vi "Create.vi"(8 "error in (no error)":errorcluster) -> (0 "error out":errorcluster, 3 "ClientPool out":refnum<class "ClientPool.lvclass">)   [LabVIEW 2020, in "MeasurementLink Measurement Server.lvlib" / "ClientPool.lvclass"]
uses:
  ClientPool.lvclass
  ClientPool.lvclass/ClientPool.ctl
  MeasurementLink Measurement Server.lvlib
  MeasurementLink Discovery Client/MeasurementLink Discovery Client.lvlib
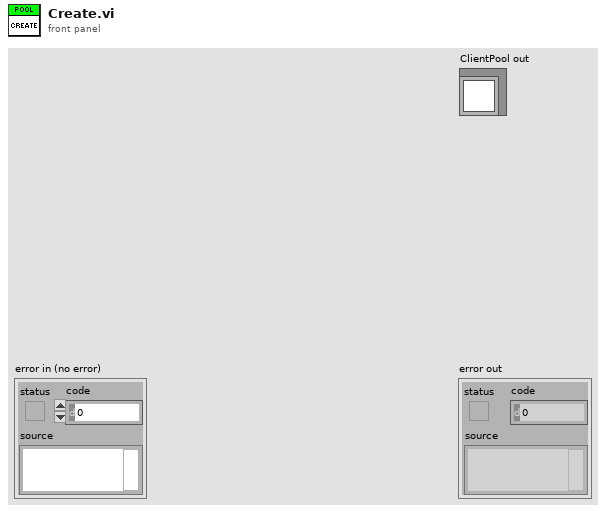
[diagram p1: front panel]
types:
  T1 = typedef "grpc-lvsupport-release.lvlib/grpcId.ctl" = u64
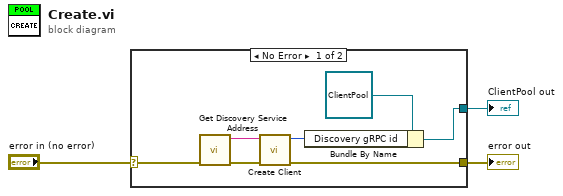
[diagram p0: block diagram]
diagram:
  n1 = case shown="No Error" "error in (no error)" {
    selector: "error in (no error)" -> [w8 w11]
    tunnel: [w7 w11] -> w2
    tunnel: [w9 _] -> w1
    frame No Error {
      n2 = call "Get Discovery Service Address.vi"("error in"=w8) -> ("error out"=w10:errorcluster, "address"=w5:string)  [unwired: 9 in]
      n3 = call "Create Client.vi"("error in"=w10, "address"=w5) -> ("error out"=w7:errorcluster, "gRPC ID Out"=w6:T1)  [unwired: 8 in]
      n4 = Bundle By Name(cluster=refnum<class "ClientPool.lvclass"> refnum ("MeasurementLink Measurement Server.lvlib:ClientPool.lvclass"), "Discovery gRPC id"=w6) -> (w9:refnum<class "ClientPool.lvclass">)
    }
    frame Error {
    }
  }
  "error out" <- w2
  "ClientPool out" <- w1
